vi "Startup.vi"   [LabVIEW 2023]
doc: "*-----------------------------------------------------\n* Author: SWatts\n*\n* VI Description: Dynamically load Splash Screen and main vi\n* \n*\n* Error handling: All errors passed out\n*\n* Pre-condition: \n*\n* Post-condition: None\n*\n* Revision History:\n*\n* Rev Date Author Description \n* 01 30/04/2014 SWatts First issue\n*\n*-----------------------------------------------------"
types:
  T1 = enum32{"Invalid", "Standard", "Closed", "Hidden", "Minimized", "Maximized"}
  T2 = enum32{"invalid app kind", "Development System", "Run Time System", "Student Edition", "Embedded LabVIEW", "Evaluation", "Custom"}
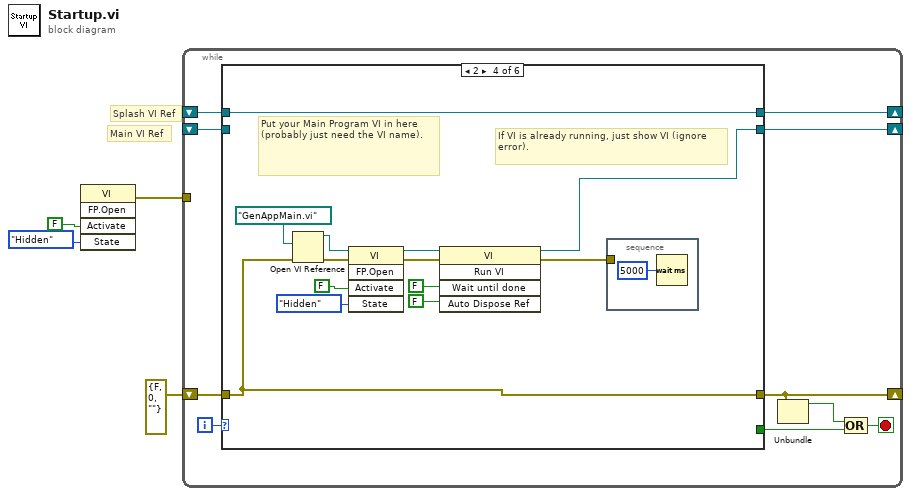
[diagram p0: block diagram]
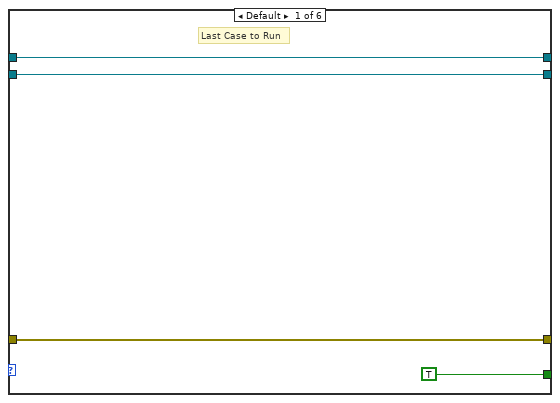
[diagram p2: hidden frame]
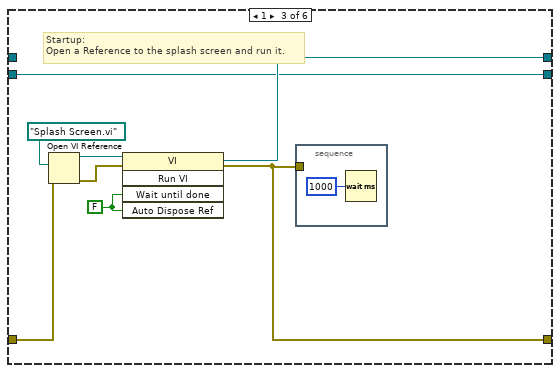
[diagram p4: hidden frame]
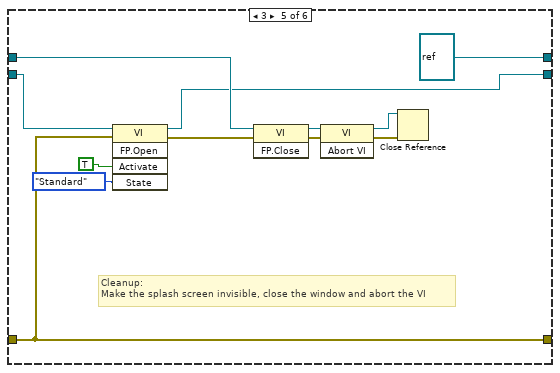
[diagram p5: hidden frame]
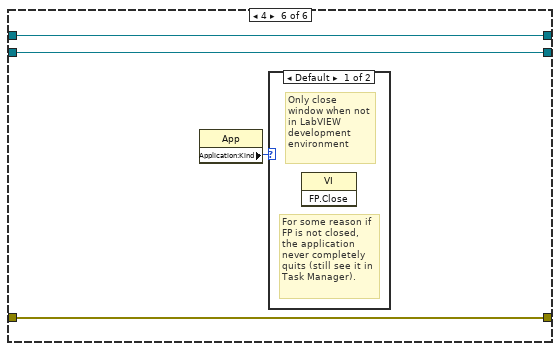
[diagram p6: hidden frame]
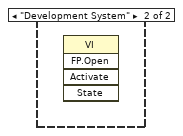
[diagram p7: hidden frame]
diagram:
  # "Main VI Ref"
  # "Splash VI Ref"
  n1 = invoke class="VI" method="FP.Open"("Activate"=FALSE ("Activate?"), "State"=T1."Hidden") -> (error out=w1:errorcluster)  [unwired: 3 in, 4 out]
  n2 = while {
    shift-right: [w7] -> _
    shift-left: errorcluster {"status"=FALSE, "code"=0, "source"=""} ("error out") -> [w8]
    shift-right: [w10] -> _
    shift-left: _ -> [w9]
    tunnel: w1 -> [_]
    shift-right: [w6] -> _
    shift-left: _ -> [w5]
    i -> [w14]
    stop <- w12 stop-if-true
    n3 = case shown="2" w14 {
      tunnel: [TRUE _ _ _ _ _] -> w13
      tunnel: [w17 w21 w28 w40 refnum<vi> refnum w59] -> w10
      tunnel: w9 -> [w17 w21 _ w40 w51 w59]
      tunnel: w8 -> [w16 w20 w27 w39 w49 w58]
      tunnel: [w16 w20 w26 w39 w49 w58] -> w7
      tunnel: [w15 w19 w22 w32 w45 w57] -> w6
      tunnel: w5 -> [w15 w19 w22 _ w47 w57]
      frame Default {
        # "Last Case to Run"
      }
      frame 0 {
        # "Initialize Case - might not be needed."
      }
      frame 1 {
        w25 = FALSE ("Wait Until Done")
        # "Startup:\nOpen a Reference to the splash screen and run it."
        n4 = Open VI Reference(vi path=path "Splash Screen.vi", error in (no error)=w27) -> (vi reference=w24:refnum<vi>, error out=w23:errorcluster)  [unwired: 4 in]
        n5 = invoke class="VI" method="Run VI"(reference=w24, error in=w23, "Wait until done"=w25, "Auto Dispose Ref"=w25) -> (reference out=w28:refnum<vi>, error out=w26:errorcluster)  [unwired: 1 in, 3 out]
        n6 = stacked-sequence {
          tunnel: w26 -> [_]
          frame #0 {
            n7 = Wait (ms)(milliseconds to wait=u32 1000) -> ()  [unwired: 1 out]
          }
        }
      }
      frame 2 {
        # "Put your Main Program VI in here (probably just need the VI name)."
        # "If VI is already running, just show VI (ignore error)."
        n8 = Open VI Reference(vi path=path "GenAppMain.vi", error in (no error)=w39) -> (vi reference=w36:refnum<vi>, error out=w34:errorcluster)  [unwired: 4 in]
        n9 = invoke class="VI" method="FP.Open"(reference=w36, error in=w34, "Activate"=FALSE ("Activate?"), "State"=T1."Hidden") -> (reference out=w35:refnum<vi>, error out=w33:errorcluster)  [unwired: 1 in, 3 out]
        n10 = invoke class="VI" method="Run VI"(reference=w35, error in=w33, "Wait until done"=FALSE ("Wait Until Done"), "Auto Dispose Ref"=FALSE ("Auto Dispose Reference")) -> (reference out=w32:refnum<vi>, error out=w31:errorcluster)  [unwired: 1 in, 3 out]
        n11 = stacked-sequence {
          tunnel: w31 -> [_]
          frame #0 {
            n12 = Wait (ms)(milliseconds to wait=u32 5000) -> ()  [unwired: 1 out]
          }
        }
      }
      frame 3 {
        # "Cleanup:\nMake the splash screen invisible, close the window and abort the VI"
        n13 = invoke class="VI" method="FP.Open"(reference=w47, error in=w49, "Activate"=TRUE ("Activate?"), "State"=T1."Standard") -> (reference out=w45:refnum<vi>, error out=w46:errorcluster)  [unwired: 1 in, 3 out]
        n14 = invoke class="VI" method="FP.Close"(reference=w51, error in=w46) -> (reference out=w54:refnum<vi>, error out=w53:errorcluster)  [unwired: 1 in, 1 out]
        n15 = invoke class="VI" method="Abort VI"(reference=w54, error in=w53) -> (reference out=w56:refnum<vi>, error out=w55:errorcluster)  [unwired: 1 in, 1 out]
        n16 = Close Reference(reference=w56, error in (no error)=w55) -> ()  [unwired: 1 out]
      }
      frame 4 {
        n17 = property class="App"() -> ("Application:Kind"=w60:T2)  [unwired: 2 in, 2 out]
        n18 = case shown="Default" w60 {
          frame Default {
            # "For some reason if FP is not closed, the application never completely quits (still see it in Task Manager)."
            # "Only close window when not in LabVIEW development environment"
            n19 = invoke class="VI" method="FP.Close"() -> ()  [unwired: 3 in, 3 out]
          }
          frame "Development System" {
            n20 = invoke class="VI" method="FP.Open"() -> ()  [unwired: 5 in, 5 out]
          }
        }
      }
    }
    n21 = Unbundle(w7) -> ("status"=w11:bool)  [unwired: 2 out]
    n22 = Compound Arithmetic op=OR(w11, w13) -> (w12:bool)
  }
